vi "Get WIFI SSID.vi"(8 "Error In":errorcluster, 11 "LINX Device Config":T1) -> (0 "Error Out":errorcluster, 2 "SSID":string, 3 "LINX Device Config":T1)   [LabVIEW 2011, in "LVH-LINX.lvlib" / "Device.lvlib"]
uses:
  Device.lvlib
  Type Defs/LINX Device Config.ctl
  Type Defs/Interface.ctl
  Type Defs/TCP Config.ctl
  Type Defs/Device Family.ctl
  Type Defs/Channels.ctl
  Type Defs/Error Type.ctl
  LVH-LINX.lvlib
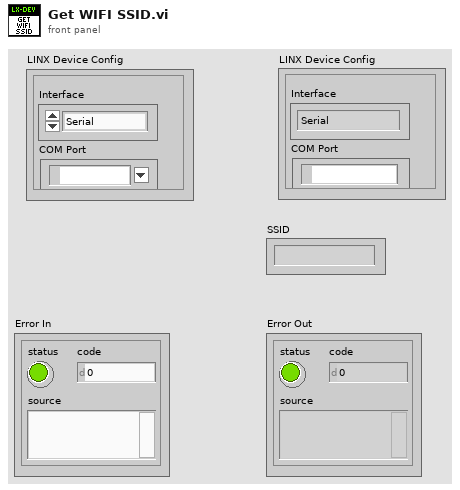
[diagram p1: front panel]
types:
  T1 = typedef "LVH-LINX.lvlib/Device.lvlib/LINX Device Config.ctl" = cluster{"Interface":T2, "COM Port":refnum<visa-resource-name>, "TCP Configuration":T3, "Device Family":T4, "Device ID":u8, "Device Name":string, "TCP Ref":refnum<k5>, "Channels":T5}
  T2 = typedef "LVH-LINX.lvlib/Interface.ctl" = enum16{"Serial", "TCP"}
  T3 = typedef "LVH-LINX.lvlib/Device.lvlib/TCP Config.ctl" = cluster{"IP Address":string, "Port":u16}
  T4 = typedef "LVH-LINX.lvlib/Device Family.ctl" = enum8{"National Instruments", "Digilent", "Arduino"}
  T5 = typedef "LVH-LINX.lvlib/Channels.ctl" = cluster{"DI Channels":u8[], "DO Channels":u8[], "AI":u8[], "AO":u8[], "PWM":u8[], "QE":u8[], "UART":u8[], "I2C 2":u8[], "SPI":u8[], "CAN":u8[], "AI Ref (V)":dbl, "AO Resolution (Bits)":u8, "AO Ref (V)":dbl}
  T6 = typedef "LVH-LINX.lvlib/Error Type.ctl" = enum16{"Unknown", "Timeout", "Corrupt Return Packet", "Unable To Connect", "Command Not Supported", "Channel DNE", "Invalid COM Config"}
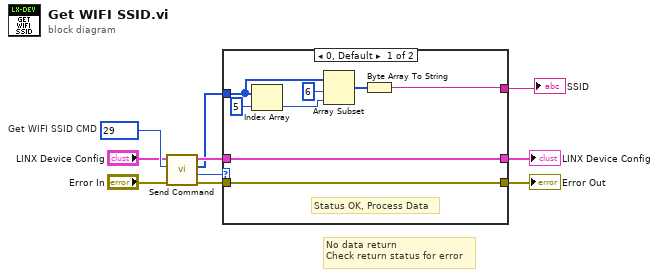
[diagram p0: block diagram]
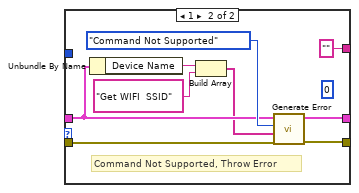
[diagram p2: hidden frame]
diagram:
  w9 = u16 29  # Get WIFI SSID CMD
  # "No data return\nCheck return status for error"
  n1 = call "Send Command.vi"("Error In"="Error In", "CMD"=w9, "LINX Device Config"="LINX Device Config") -> ("Error Out"=w4:errorcluster, "Status"=w2:u8, "Response"=w3:u8[], "LINX Device Config"=w6:T1)  [unwired: 5 in]
  n2 = case shown="0, Default" w2 {
    tunnel: [w17 w25] -> w7
    tunnel: w6 -> [w17 w21]
    tunnel: [w18 w26] -> w5
    tunnel: w4 -> [w18 w27]
    tunnel: w3 -> [w15 _]
    tunnel: [w11 "" ("string")] -> w1
    frame 0, Default {
      # "Status OK, Process Data"
      n3 = Index Array(array=w15, index=5) -> (element=w13:u8)
      n4 = Array Subset(array=w15, index=6, length=w13) -> (w12:u8[])
      n5 = Byte Array To String(unsigned byte array=w12) -> (string=w11:string)
    }
    frame 1 {
      (unwired) u16 0
      # "Command Not Supported, Throw Error"
      n6 = Unbundle By Name(w21) -> ("Device Name"=w22:string)
      n7 = Build Array(w22, "Get WIFI  SSID") -> (w20:string[])
      n8 = call "Generate Error.vi"("Error In"=w27, "Arguments"=w20, "Error Type"=Error_Type."Command Not Supported", "LINX Device Config"=w21) -> ("Error Out"=w26:errorcluster, "LINX Device Config"=w25:T1)  [unwired: 6 in]
    }
  }
  "Error Out" <- w5
  "LINX Device Config" <- w7
  "SSID" <- w1
